vi "WheelAvg.vi"(8 "Calculate Rotation?":bool, 9 "Robot Angle (degrees)":dbl(knob) scale=180.0..-180.0, 10 "wheel Y movements (FL, FR, RL, RR)":dbl[](array[numeric]), 11 "wheel X movements (FL, FR, RL, RR)":dbl[](array[numeric])) -> (1 "Rotation":dbl, 2 "Y":dbl, 3 "X":dbl)   [LabVIEW 2014, in "Team900SwerveDrive.lvlib"]
uses:
  Team900SwerveDrive.lvlib
  <vilib>/Analysis/baseanly.llb/Mean (DBL).vi
  SwerveGlobalData.vi
  <vilib>/Analysis/NI_AALBase.lvlib
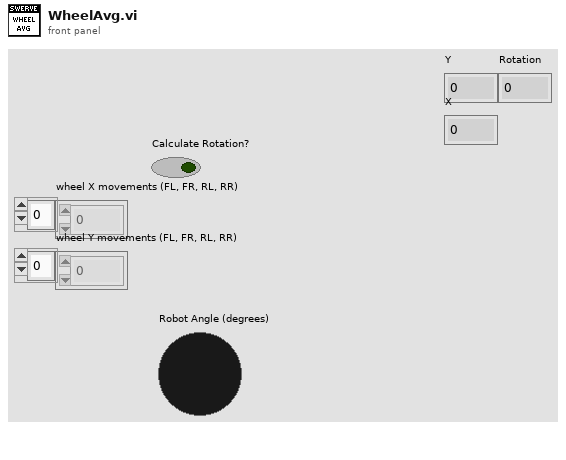
[diagram p1: front panel]
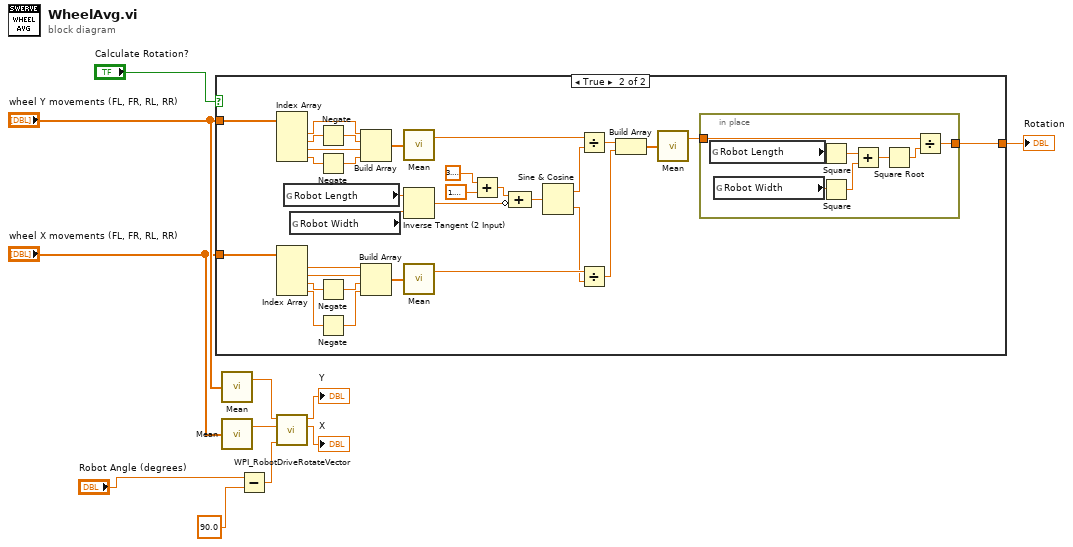
[diagram p0: block diagram]
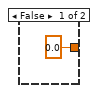
[diagram p2: hidden frame]
diagram:
  n1 = case shown="True" "Calculate Rotation?" {
    tunnel: [0.0 ("mean") w13] -> w11
    tunnel: "wheel Y movements (FL, FR, RL, RR)" -> [_ w28]
    tunnel: "wheel X movements (FL, FR, RL, RR)" -> [_ w25]
    frame False {
    }
    frame True {
      n2 = Index Array(array=w28) -> (element #1=w21:dbl, element #2=w27:dbl, element #3=w23:dbl, element #4=w26:dbl)  [unwired: 4 in]
      n3 = Index Array(array=w25) -> (element #1=w15:dbl, element #2=w16:dbl, element #3=w20:dbl, element #4=w19:dbl)  [unwired: 4 in]
      n4 = global read "SwerveGlobalData.vi" "Robot Length"() -> (w34:dbl)
      n5 = global read "SwerveGlobalData.vi" "Robot Width"() -> (w35:dbl)
      n6 = Negate(x=w27) -> (-x=w22:dbl)
      n7 = Negate(x=w26) -> (-x=w24:dbl)
      n8 = Negate(x=w20) -> (-x=w18:dbl)
      n9 = Negate(x=w19) -> (-x=w17:dbl)
      n10 = Build Array(w21, w22, w23, w24) -> (w43:dbl[])
      n11 = Build Array(w15, w16, w18, w17) -> (w41:dbl[])
      n12 = call-poly <vilib>:"Mean.vi"("X"=w43) -> ("mean"=w42:dbl)  [unwired: 1 out]
      n13 = Inverse Tangent (2 Input)(1:w35, 2:w34) -> (0:w36:dbl)
      n14 = call-poly <vilib>:"Mean.vi"("X"=w41) -> ("mean"=w40:dbl)  [unwired: 1 out]
      n15 = Add(x=3.141592653589793, y=1.5707963267948966) -> (x+y=w37:dbl)
      n16 = Compound Arithmetic op=ADD(w37, invert w36) -> (w33:dbl)
      n17 = Sine & Cosine(0:w33) -> (1:w29:dbl, 2:w30:dbl)
      n18 = Divide(x=w42, y=w29) -> (x/y=w31:dbl)
      n19 = Divide(x=w40, y=w30) -> (x/y=w32:dbl)
      n20 = Build Array(w31, w32) -> (w44:dbl[])
      n21 = call-poly <vilib>:"Mean.vi"("X"=w44) -> ("mean"=w14:dbl)  [unwired: 1 out]
      n22 = in-place {
        in-place-border: w14 -> [w46]
        in-place-border: [w45] -> w13
        n23 = global read "SwerveGlobalData.vi" "Robot Length"() -> (w52:dbl)
        n24 = global read "SwerveGlobalData.vi" "Robot Width"() -> (w51:dbl)
        n25 = Square(x=w52) -> (x^2=w49:dbl)
        n26 = Square(x=w51) -> (x^2=w50:dbl)
        n27 = Add(x=w49, y=w50) -> (x+y=w48:dbl)
        n28 = Square Root(x=w48) -> (sqrt(x)=w47:dbl)
        n29 = Divide(x=w46, y=w47) -> (x/y=w45:dbl)
      }
    }
  }
  "Rotation" <- w11
  n30 = call-poly <vilib>:"Mean.vi"("X"="wheel Y movements (FL, FR, RL, RR)") -> ("mean"=w5:dbl)  [unwired: 1 out]
  n31 = call-poly <vilib>:"Mean.vi"("X"="wheel X movements (FL, FR, RL, RR)") -> ("mean"=w8:dbl)  [unwired: 1 out]
  n32 = Subtract(x="Robot Angle (degrees)", y=90.0 ("x")) -> (x-y=w9:dbl)
  n33 = call <vilib>:"WPI_RobotDriveRotateVector.vi"("Angle"=w9, "X"=w8, "Y"=w5) -> ("X'"=→"X":dbl, "Y'"=→"Y":dbl)  [unwired: 7 out]
